vi "Panel-NicmosPiezo.vi"() -> ()   [LabVIEW 2009]
uses:
  <vilib>/Analysis/2dsp.llb/Power Spectrum (DBL).vi
  <vilib>/Analysis/NI_AALBase.lvlib
  <vilib>/Analysis/NI_AALPro.lvlib
panel:
  out "Contraste":dbl(graph)=1.1290322580645162
  in  "Filter":bool=TRUE
  out "Flux":dbl(graph)=15.198039215686274
  in  "Filter length 2":i32=150
  in  "Starting index 2":i32=175
  in  "Filter length 1":i32=75
  in  "Starting index 1":i32=2
  in  "Commande onglet":T1(tab)
  out "Std Dev 2":dbl=38.11590970376363 format="%.1f"
  out "Std Dev":dbl=6.173808363057897 format="%.1f"
  in  "Integrate pattern":bool=TRUE
  out "Mean Level":dbl=15.198039215686274 format="%.1f"
  out "Total NRJ":i32=7797
  out "Scan":i32[](graph)=[11, 26, 19, 3, 17, 23, 6, 12, 24, 14, 15, 19, 7, 11, 25, 19, 12, 12, 11, 16, 21, 18, 13, 8, 14, 23, 16, 10, 16, 12, 14, 24, 12, 3, 20, 21, 11, 14, 12, 13, 23, 13, 7, 22, 17, 7, 20, 18, 6, 17, 24, 11, 9, 15, 17, 18, 15, 12, 13, 13, 16, 20, 13, 8, 14, 19, 16, 11, 11, 17, 18, 13, 11, 12, 18, 19, 9, 9, 22, 17, 5, 15, 23, 10, 10, 20, 14, 6, 17, 23, 10, 7, 18, 18, 10, 12, 18, 16, 10, 10, 19, 18, 6, 12, 25, 12, 2, 19, 21, 10, 13, 13, 10, 17, 16, 12, 17, 10, 9, 24, 17, 1, 15, 24, 13, 10, 13, 13, 19, 16, 9, 15, 16, 9, 15, 21, 12, 8, 17, 18, 6, 11, 26, 15, 1, 15, 24, 10, 10, 18, 16, 13, 10, 11, 19, 19, 12, 11, 9, 13, 26, 17, 0, 13, 25, 12, 8, 16, 19, 15, 10, 13, 19, 12, 9, 17, 19, 15, 10, 5, 17, 30, 12, -2, 14, 25, 16, 8, 12, 19, 14, 10, 21, 15, 3, 20, 26, 5, 9, 22, 11, 15, 23, 4, 8, 29, 14, 1, 19, 25, 10, 7, 17, 20, 12, 11, 19, 15, 7, 17, 20, 11, 16, 18, 8, 11, 22, 16, 9, 18, 19, 9, 12, 23, 15, 7, 20, 20, 6, 15, 23, 11, 14, 21, 8, 9, 25, 19, 9, 13, 15, 17, 20, 13, 11, 16, 17, 14, 14, 16, 13, 12, 23, 22, 0, 7, 33, 20, 3, 15, 14, 11, 27, 18, 1, 17, 23, 12, 16, 17, 11, 17, 17, 13, 18, 17, 15, 16, 8, 18, 30, 7, 2, 30, 20, 2, 22, 23, 3, 16, 25, 13, 15, 15, 9, 20, 24, 13, 8, 12, 21, 26, 12, 6, 18, 21, 18, 20, 9, 6, 25, 25, 9, 10, 17, 17, 20, 16, 9, 14, 22, 19, 13, 12, 18, 22, 12, 11, 23, 17, 5, 18, 27, 11, 10, 24, 15, 8, 24, 24, 7, 14, 23, 10, 14, 30, 15, -1, 20, 31, 12, 6, 21, 22, 10, 15, 23, 13, 13, 23, 16, 9, 19, 19, 14, 19, 16, 14, 23, 15, 7, 22, 21, 11, 20, 16, 6, 23, 25, 9, 17, 21, 8, 18, 26, 13, 15, 16, 9, 22, 26, 7, 12, 25, 16, 12, 16, 18, 21, 15, 9, 21, 20, 9, 18, 21, 12, 15, 17, 15, 21, 16, 10, 21, 20, 9, 15, 23, 19, 14, 11, 18, 22, 11, 16, 28, 12, 3, 23, 28, 14, 8, 12, 24, 23, 7, 11, 25, 16, 11, 20, 17, 15, 16, 13, 21, 23, 5, 12, 28, 13, 8, 23, 18, 10, 14, 18, 21, 16, 8, 19, 24, 8, 9, 26, 21, 10, 10, 17, 23, 17, 7, 17, 25, 11, 7, 19, 20, 14, 18, 18, 7, 10, 27, 23, 8, 14, 17, 9, 20, 27, 8, 5, 23, 20, 9, 13, 21, 22, 12]
  out "Image":i32[][](graph)=[[8, -3, -1], [3, 4, 5], [1, 4, 2]]
  out "Power Spectrum":cluster{dbl[unit][], "Power Spectrum":dbl[]}(graph)
  in  "noise":bool=TRUE
  out "fringes":bool
  in  "filtre maxima (%)":dbl(slide)=0.10204081632653061 scale=0.0..10.0
  out "2 polarizations 2":i32[][](graph)=[[652, 1046, 953], [663, 1272, 1188], [405, 872, 746]]
  out "y":dbl=0.7916666666666666 format="%.1f"
  out "x":dbl=0.9583333333333334 format="%.1f"
  out "b":dbl=1.1104675703322058 format="%.2f"
  out "theta":dbl[unit]=0.06900301182875972 format="%.2f"
  out "a":dbl=0.8351591910897948 format="%.2f"
  out "Graphe d'intensité 2":i32[][](graph)=[[29, 34, 27], [35, 42, 30], [22, 33, 19]]
  out "Y":dbl format="%.2f"
  out "X":dbl format="%.2f"
  out "Waist  Y":dbl format="%.2f"
  out "Waist  X":dbl format="%.2f"
  out "Cut X":i32[](graph)=[11, 8, 2]
  out "Cut Y":i32[](graph)=[11, 8, 6]
  out "TF":dbl[](graph)
  out "Vertical cut":dbl[](graph)
  out "DSP":cluster{dbl[unit][], "Power Spectrum":dbl[]}(graph)
  in  "RESET ACCUMULATE":bool
  in  "RESET ACCUMULATE 2":bool
  out "Graphe XY":cluster{dbl[], dbl[]}(graph)={[1341175.125, 1343537.125, 1345374.5, 1349276.0, 1353395.625, 1355804.625, 1356299.25, 1315217.375, 1314825.25], [2425317.4836309524, 2730754.322916748, 3781664.8095238847, 1635464.059523804, 5468045.299107264, 1983356.644345304, 2776568.125, 1310442574.483631, 1184346966.910715]}
  out "Standard Deviation":dbl(graph)=100014.63289358855
  in  "Filter?":bool
  out "Graphe XY 2":cluster{dbl[unit][], "Power Spectrum":dbl[]}(graph)={[0.0, 5.7230419684975145, 11.446083936995029, 17.169125905492542, 22.892167873990058, 28.615209842487573, 34.338251810985085, 40.0612937794826], "Power Spectrum"=[1732307746455.1406, 2670579822.32282, 1023845913.265625, 501399858.4584302, 360909755.640625, 501399858.4584302, 1023845913.265625, 2670579822.32282]}
  out "Graphe":dbl[](graph)=[1505710.0, 1422929.0, 1333372.0, 1291362.0, 1266016.0, 1249535.0, 1235579.0, 1224870.0]
  in  "Freq":dbl[](array[numeric])
  out "Time":dbl[unit]=2.4961750000000003e-06
  out "Graphe 2":i32[](graph)
  in  "Image index":i32
  in  "STOP":bool
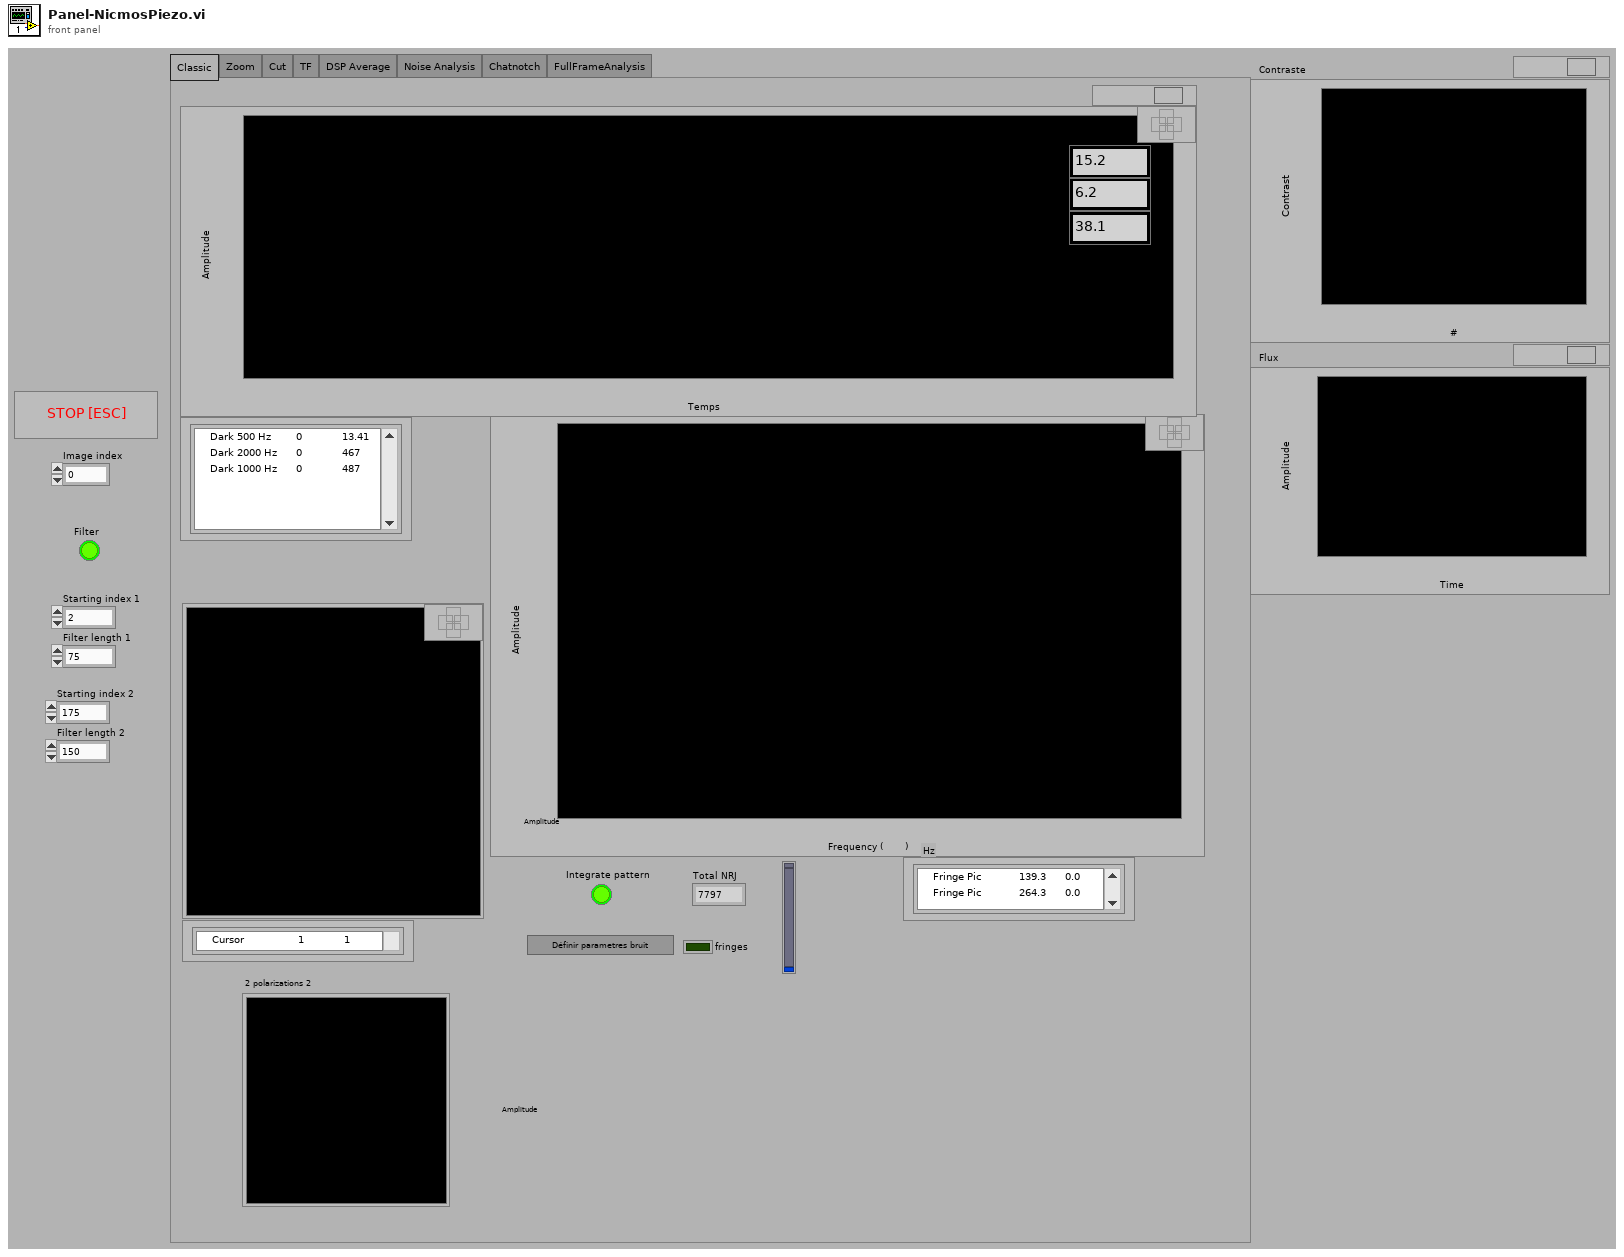
[diagram p1: front panel]
types:
  T1 = enum32{"Classic", "Zoom", "Cut", "TF", "DSP Average", "Noise Analysis", "Chatnotch", "FullFrameAnalysis"}
  T2 = typedef "NICMOS.READOUT.ctl" = cluster{"Readout":i32, "Deglitch":i32, "Framerate":dbl[unit], "Bank":i32}
  T3 = typedef "NICMOS.DATA.ctl" = cluster{"DATA":i32[][][], "INDEX":i32}
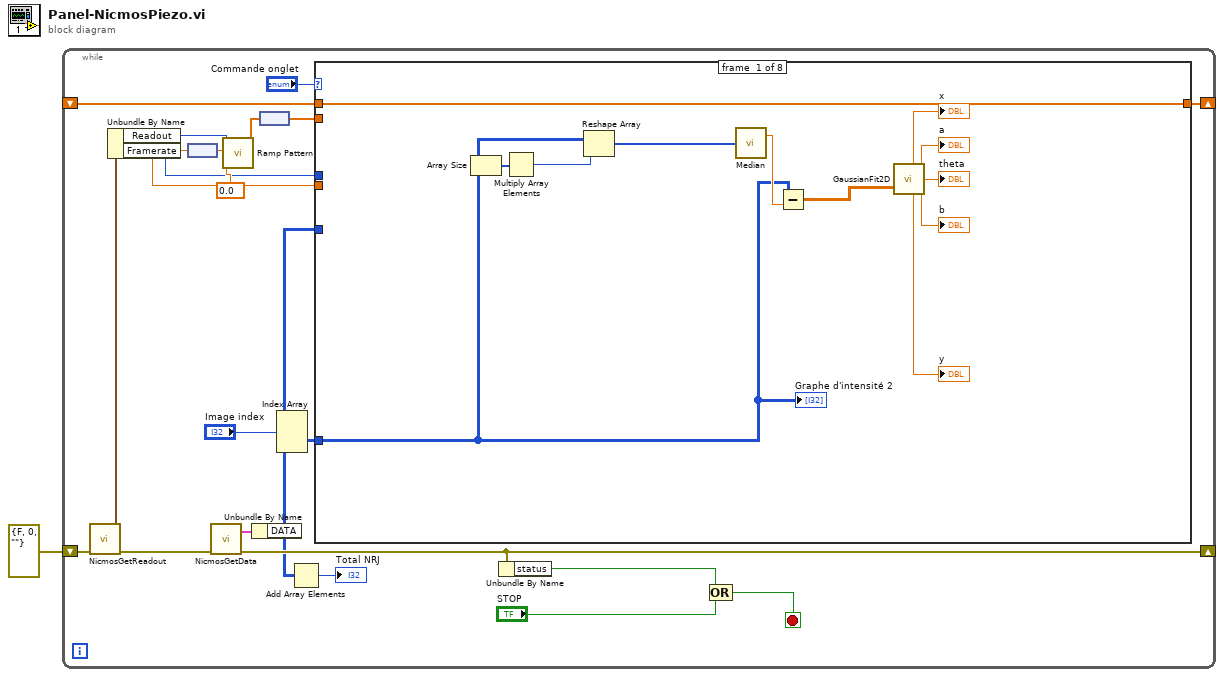
[diagram p0: block diagram]
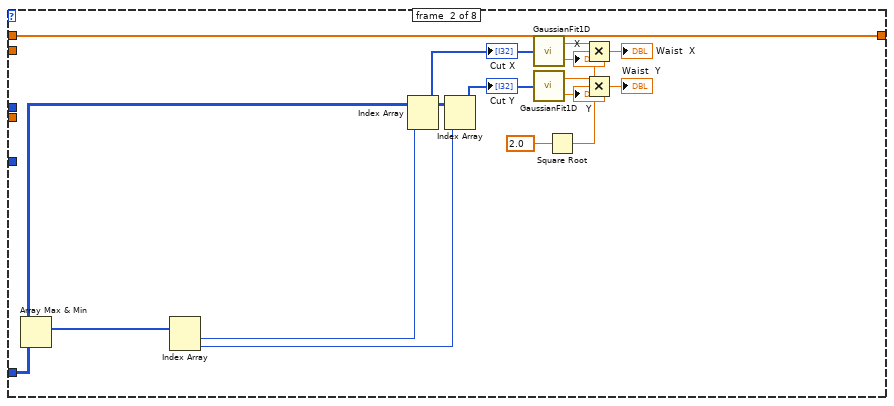
[diagram p2: hidden frame]
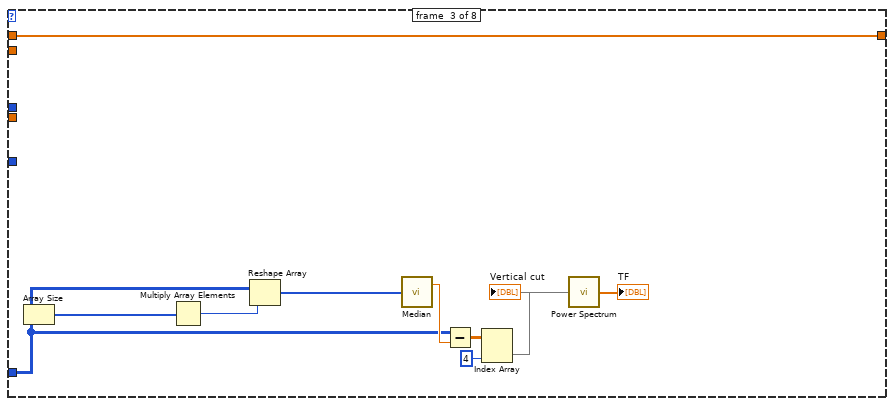
[diagram p3: hidden frame]
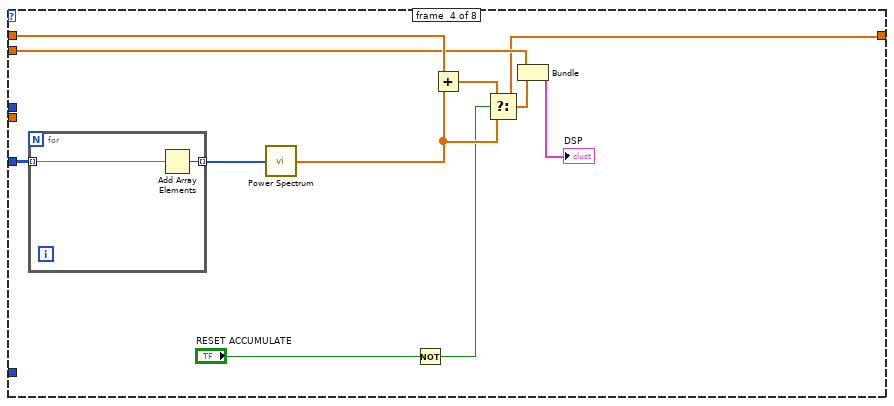
[diagram p4: hidden frame]
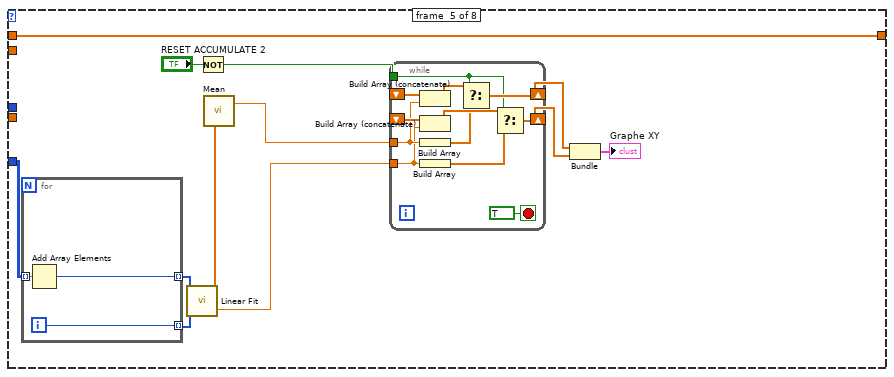
[diagram p5: hidden frame]
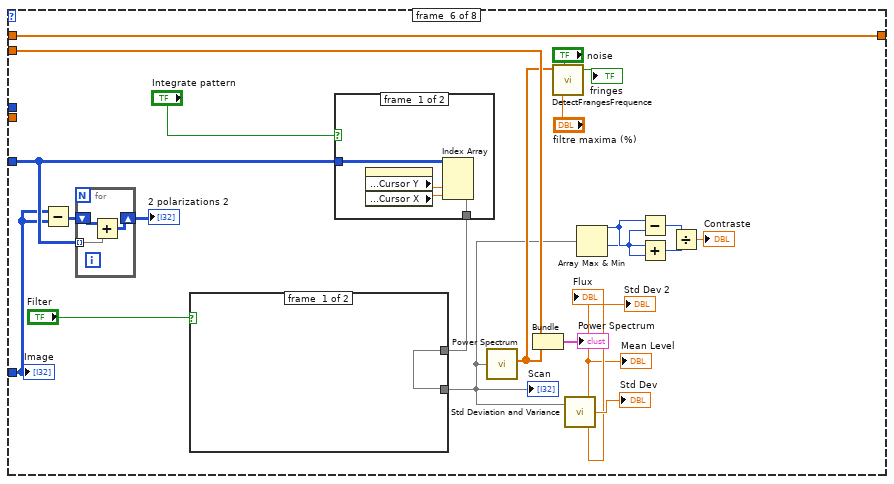
[diagram p6: hidden frame]
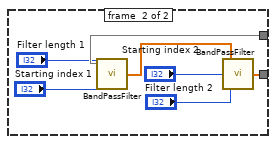
[diagram p7: hidden frame]
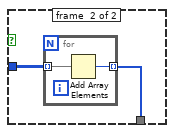
[diagram p8: hidden frame]
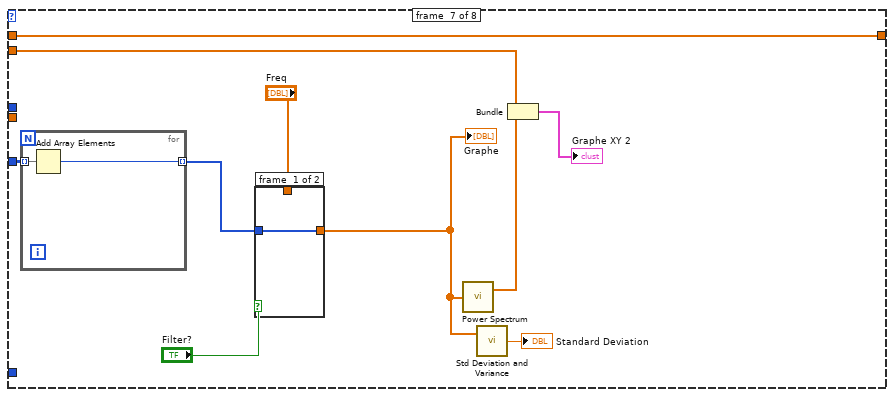
[diagram p9: hidden frame]
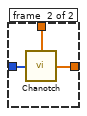
[diagram p10: hidden frame]
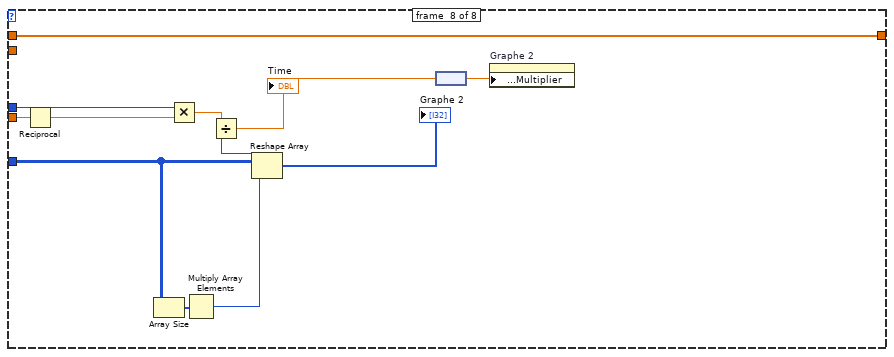
[diagram p11: hidden frame]
diagram:
  n1 = while {
    shift-left: errorcluster {"status"=FALSE, "code"=0, "source"=""} ("error out") -> [w10]
    shift-right: [w16] -> _
    shift-right: [w14] -> _
    shift-left: _ -> [w15]
    stop <- w11 stop-if-true
    n2 = call "NicmosGetReadout.vi"("error in (no error)"=w10) -> ("READOUT out"=w5:T2, "error out"=w9:errorcluster)  [unwired: 7 in]
    n3 = Unbundle By Name(w5) -> ("Readout"=w4:i32, "Framerate"=w3:dbl[unit])
    n4 = node(w3) -> (w7:dbl)
    n5 = call "NicmosGetData.vi"("error in (no error)"=w9) -> ("DATA"=w13:T3, "error out"=w16:errorcluster)  [unwired: 7 in]
    n6 = call <vilib>:"Ramp Pattern.vi"("start"=0.0, "end"=w7, "samples"=w4) -> ("Ramp Pattern"=w8:dbl[])  [unwired: 7 in, 1 out]
    n7 = Unbundle By Name(w13) -> ("DATA"=w12:i32[][][])
    n8 = node(w8) -> (w2:dbl[unit][])
    n9 = Index Array(array=w12, index (dim 0)="Image index") -> (element=w20:i32[][])  [unwired: 2 in]
    n10 = Add Array Elements(numeric array=w12) -> (sum=→"Total NRJ":i32)
    n11 = case shown="\"Classic\", Default" "Commande onglet" {
      tunnel: w2 -> [_ _ _ w62 _ w121 w146 _]
      tunnel: w20 -> [w24 w36 w55 _ _ w105 _ _]
      tunnel: w12 -> [_ _ _ w69 w79 w106 w150 w166]
      tunnel: w15 -> [w23 w35 w50 w67 w83 w117 w147 w165]
      tunnel: [w23 w35 w50 w61 w83 w117 w147 w165] -> w14
      tunnel: w3 -> [_ _ _ _ _ _ _ w164]
      tunnel: w4 -> [_ _ _ _ _ _ _ w163]
      frame #0 {
        n12 = Array Size(array=w24) -> (size(s)=w33:i32[])
        n13 = Multiply Array Elements(1:w33) -> (0:w32:i32)
        n14 = Reshape Array(w24, w32) -> (w31:i32[])
        n15 = call <vilib>:"Median.vi"("X"=w31) -> ("median"=w29:dbl)  [unwired: 1 out]
        n16 = Subtract(x=w24, y=w29) -> (x-y=w30:dbl[][])
        n17 = call "GaussianFit2D.vi"("Image"=w30) -> ("b"=→"b":dbl, "y"=→"y":dbl, "theta"=→"theta":dbl[unit], "a"=→"a":dbl, "x"=→"x":dbl)  [unwired: 1 in]
        "Graphe d'intensité 2" <- w24
      }
      frame #1 {
        n18 = Array Max & Min(array=w36) -> (max index (indices)=w49:i32[])  [unwired: 3 out]
        n19 = Index Array(array=w49) -> (element #1=w46:i32, element #2=w47:i32)  [unwired: 2 in]
        n20 = Index Array(array=w36, index (row)=w46) -> (element=w48:i32[])  [unwired: 1 in]
        "Cut X" <- w48
        n21 = Index Array(array=w36, index (col)=w47) -> (element=w45:i32[])  [unwired: 1 in]
        "Cut Y" <- w45
        n22 = call "GaussianFit1D.vi"("Cut"=w48) -> ("Sigma"=w44:dbl, "x"=→"X":dbl)
        n23 = call "GaussianFit1D.vi"("Cut"=w45) -> ("Sigma"=w43:dbl, "x"=→"Y":dbl)
        n24 = Square Root(x=2.0) -> (sqrt(x)=w40:dbl)
        n25 = Multiply(x=w44, y=w40) -> (x*y=→"Waist  X":dbl)
        n26 = Multiply(x=w43, y=w40) -> (x*y=→"Waist  Y":dbl)
      }
      frame #2 {
        n27 = Array Size(array=w55) -> (size(s)=w59:i32[])
        n28 = Multiply Array Elements(1:w59) -> (0:w58:i32)
        n29 = Reshape Array(w55, w58) -> (w57:i32[])
        n30 = call <vilib>:"Median.vi"("X"=w57) -> ("median"=w56:dbl)  [unwired: 1 out]
        n31 = Subtract(x=w55, y=w56) -> (x-y=w54:dbl[][])
        n32 = Index Array(array=w54, index (col)=4 ("indice désactivé (col)")) -> (element=w52:dbl[])  [unwired: 1 in]
        "Vertical cut" <- w52
        n33 = call-poly <vilib>:"Power Spectrum.vi"("X"=w52) -> ("Power Spectrum"=→"TF":dbl[])  [unwired: 1 out]
      }
      frame #3 {
        n34 = for {
          tunnel: w69 -> [w71] mode=indexing
          tunnel: [w70] -> w68 mode=indexing
          n35 = Add Array Elements(numeric array=w71) -> (sum=w70:i32)
        }
        n36 = call-poly <vilib>:"Power Spectrum.vi"("X"=w68) -> ("Power Spectrum"=w65:dbl[])  [unwired: 1 out]
        n37 = Not(x="RESET ACCUMULATE") -> (.not. x?=w63:bool)
        n38 = Add(x=w67, y=w65) -> (x+y=w64:dbl[])
        n39 = Select(t=w64, s=w63, f=w65) -> (s? t:f=w61:dbl[])
        n40 = Bundle(w62, "Power Spectrum"=w61) -> (→"DSP":cluster{dbl[unit][], "Power Spectrum":dbl[]})  [unwired: 1 in]
      }
      frame #4 {
        n41 = for {
          tunnel: w79 -> [w98] mode=indexing
          tunnel: [w97] -> w75 mode=indexing
          tunnel: [w96] -> w76 mode=indexing
          i -> [w96]
          n42 = Add Array Elements(numeric array=w98) -> (sum=w97:i32)
        }
        n43 = call <vilib>:"Linear Fit.vi"("Y"=w75, "X"=w76) -> ("Best Linear Fit"=w73:dbl[], "residue"=w74:dbl)  [unwired: 9 in, 3 out]
        n44 = Not(x="RESET ACCUMULATE 2") -> (.not. x?=w77:bool)
        n45 = call <vilib>:"Mean.vi"("X"=w73) -> ("mean"=w72:dbl)  [unwired: 1 out]
        n46 = while {
          tunnel: w72 -> [w87]
          tunnel: w74 -> [w86]
          shift-right: [w93] -> w81
          shift-left: _ -> [w94]
          shift-right: [w91] -> w82
          shift-left: _ -> [w92]
          tunnel: w77 -> [w90]
          stop <- TRUE stop-if-true
          n47 = Build Array (concatenate)(w94, w87) -> (w89:dbl[])
          n48 = Build Array (concatenate)(w92, w86) -> (w88:dbl[])
          n49 = Build Array(w87) -> (w85:dbl[])
          n50 = Build Array(w86) -> (w84:dbl[])
          n51 = Select(t=w89, s=w90, f=w85) -> (s? t:f=w93:dbl[])
          n52 = Select(t=w88, s=w90, f=w84) -> (s? t:f=w91:dbl[])
        }
        n53 = Bundle(w81, w82) -> (→"Graphe XY":cluster{dbl[], dbl[]})  [unwired: 1 in]
      }
      frame #5 {
        n54 = Subtract(x=w105, y=w105) -> (x-y=w108:i32[][])
        n55 = for {
          tunnel: w106 -> [w124] mode=indexing
          shift-right: [w122] -> w107
          shift-left: w108 -> [w123]
          n56 = Add(x=w123, y=w124) -> (x+y=w122:i32[][])
        }
        "2 polarizations 2" <- w107
        n57 = case shown="True" "Integrate pattern" {
          tunnel: w106 -> [w135 w138]
          tunnel: [w134 w137] -> w111
          frame #0 {
            n58 = property on="Image" class="GraphIntens (strict)"() -> ("Cursor.Cursor Position:Cursor Y"=w136:dbl, "Cursor.Cursor Position:Cursor X"=w133:dbl)  [unwired: 2 in, 2 out]
            n59 = Index Array(array=w135, index (dim 1)=w136, index (dim 2)=w133) -> (element=w134:i32[])  [unwired: 1 in]
          }
          frame #1 {
            n60 = for {
              tunnel: w138 -> [w140] mode=indexing
              tunnel: [w139] -> w137 mode=indexing
              n61 = Add Array Elements(numeric array=w140) -> (sum=w139:i32)
            }
          }
        }
        n62 = case shown="True" "Filter" {
          tunnel: w111 -> [w125 w132]
          tunnel: [w125 w127] -> w99
          frame #0 {
          }
          frame #1 {
            n63 = call "BandPassFilter.vi"("Filter length"="Filter length 1", "Starting index"="Starting index 1", "CAID sequence"=w132) -> ("Filtered CAID sequence"=w126:dbl[])
            n64 = call "BandPassFilter.vi"("Filter length"="Filter length 2", "Starting index"="Starting index 2", "CAID sequence"=w126) -> ("Filtered CAID sequence"=w127:dbl[])
          }
        }
        "Scan" <- w99
        n65 = call-poly <vilib>:"Power Spectrum.vi"("X"=w99) -> ("Power Spectrum"=w110:dbl[])  [unwired: 1 out]
        n66 = Bundle(w121, "Power Spectrum"=w110) -> (→"Power Spectrum":cluster{dbl[unit][], "Power Spectrum":dbl[]})  [unwired: 1 in]
        n67 = call "DetectFrangesFrequence.vi"("spectre de frequence"=w110, "filtre maxima (%)"="filtre maxima (%)", "c'est du bruit"="noise") -> ("frange"=→"fringes":bool)  [unwired: 3 in, 1 out]
        n68 = call <vilib>:"Std Deviation and Variance.vi"("X"=w99) -> ("mean"=→"Mean Level" →"Flux":dbl, "standard deviation"=→"Std Dev":dbl, "variance"=→"Std Dev 2":dbl)  [unwired: 1 in]
        n69 = Array Max & Min(array=w99) -> (max value=w102:i32, min value=w101:i32)  [unwired: 2 out]
        n70 = Subtract(x=w102, y=w101) -> (x-y=w104:i32)
        n71 = Add(x=w102, y=w101) -> (x+y=w103:i32)
        n72 = Divide(x=w104, y=w103) -> (x/y=→"Contraste":dbl)
        "Image" <- w105
      }
      frame #6 {
        n73 = for {
          tunnel: w150 -> [w156] mode=indexing
          tunnel: [w155] -> w149 mode=indexing
          n74 = Add Array Elements(numeric array=w156) -> (sum=w155:i32)
        }
        n75 = case shown="False" "Filter?" {
          tunnel: w149 -> [w151 w154]
          tunnel: "Freq" -> [_ w153]
          tunnel: [w151 w152] -> w142
          frame #0 {
          }
          frame #1 {
            n76 = call "Chanotch.vi"("Signal"=w154, "Freq"=w153) -> ("Chanotched Signal"=w152:dbl[])
          }
        }
        "Graphe" <- w142
        n77 = call-poly <vilib>:"Power Spectrum.vi"("X"=w142) -> ("Power Spectrum"=w145:dbl[])  [unwired: 1 out]
        n78 = call <vilib>:"Std Deviation and Variance.vi"("X"=w142) -> ("standard deviation"=→"Standard Deviation":dbl)  [unwired: 1 in, 2 out]
        n79 = Bundle(w146, "Power Spectrum"=w145) -> (→"Graphe XY 2":cluster{dbl[unit][], "Power Spectrum":dbl[]})  [unwired: 1 in]
      }
      frame #7 {
        n80 = Reciprocal(x=w164) -> (1/x=w162:dbl[unit])
        n81 = Array Size(array=w166) -> (size(s)=w167:i32[])
        n82 = Multiply(x=w163, y=w162) -> (x*y=w160:dbl[unit])
        n83 = Multiply Array Elements(1:w167) -> (0:w159:i32)
        n84 = Divide(x=w160, y=w159) -> (x/y=w158:dbl[unit])
        "Time" <- w158
        n85 = Reshape Array(w166, w159) -> (→"Graphe 2":i32[])
        n86 = node(w158) -> (w157:dbl)
        n87 = property on="Graphe 2" class="GrapheWaveform (strict)"("X Scale.Offset and Multiplier:Multiplier"=w157) -> ()  [unwired: 2 in, 2 out]
      }
    }
    n88 = Unbundle By Name(w16) -> ("status"=w22:bool)
    n89 = Compound Arithmetic op=OR(w22, "STOP") -> (w11:bool)
  }
